vi "Degrees to Radians (Array EXT).vi"(3 "angles (deg)":ext[](array[numeric])) -> (1 "angles (rad)":ext[](array[numeric]))   [LabVIEW 2020, in "NI_AngleManipulation.lvlib"]
doc: "Converts a 1D array of angles from degrees to radians."
uses:
  <vilib>/Utility/AngleManip/NI_AngleManipulation.lvlib
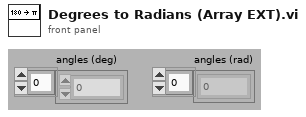
[diagram p1: front panel]
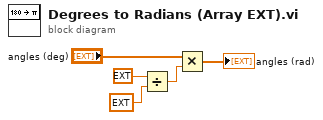
[diagram p0: block diagram]
diagram:
  n1 = Divide(x=ext 3.1415926535897932385, y=ext 180.0) -> (x/y=w3:ext)
  n2 = Multiply(x="angles (deg)", y=w3) -> (x*y=→"angles (rad)":ext[])
